vi "Get Impedance Meas Value.vi"(8 "error in (no error)":errorcluster, 11 "VISA resource name":refnum<visa-resource-name>) -> (0 "error out":errorcluster, 1 "Value Units":i32, 2 "Meas Value":dbl format="%^.3e", 3 "VISA resource name out":refnum<visa-resource-name>)   [LabVIEW 2013, in "Fluke 5XXX Series Multicalibrators.lvlib"]
doc: "This VI returns the last value of the scope impedance measurement. The unit returns indicates the status of the reading. Returns 0 and NONE when there is no recent measurement either because the Calibrator is not in a measurement mode, or because no measurement has been made yet.\n\nNote:\n\nThis VI is available only for instrument models 5500A and 5520A with oscilloscope option SC600 (SC1100)."
uses:
  Fluke 5XXX Series Multicalibrators.lvlib
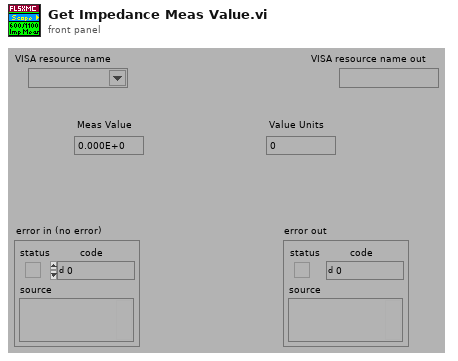
[diagram p1: front panel]
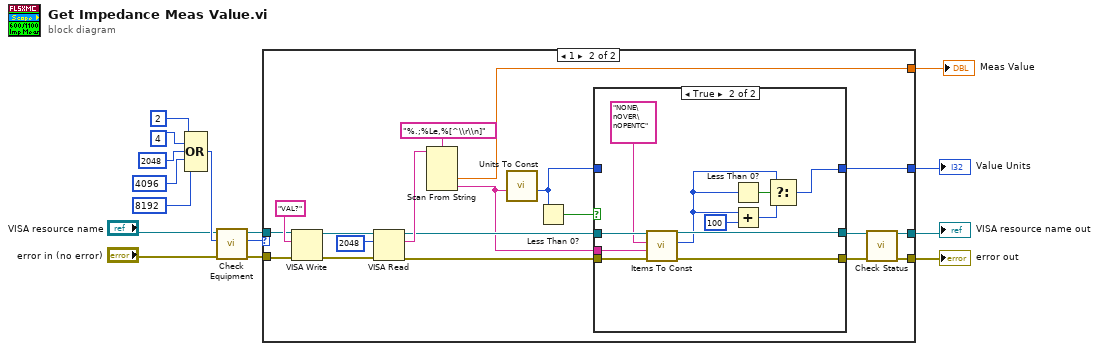
[diagram p0: block diagram]
diagram:
  n1 = Compound Arithmetic op=OR(2 ("Numeric"), 4 ("Numeric"), 2048 ("Numeric"), 4096 ("Numeric"), 8192 ("Numeric")) -> (w10:i32)
  n2 = call "Check Equipment.vi"("error in (no error)"="error in (no error)", "Bit Mask"=w10, "VISA resource name"="VISA resource name") -> ("error out"=w6:errorcluster, "Present?"=w5:u32, "VISA resource name out"=w7:refnum<visa-resource-name>)  [unwired: 6 in]
  n3 = case shown="1" w5 {
    tunnel: [w19 w33] -> w3
    tunnel: [w16 w32] -> w4
    tunnel: w6 -> [w19 w34]
    tunnel: [0.0 w29] -> w1
    tunnel: [0 w27] -> w2
    tunnel: w7 -> [w16 w21]
    frame 0, Default {
    }
    frame 1 {
      n4 = VISA Write(VISA resource name=w21, write buffer="VAL?", error in (no error)=w34) -> (VISA resource name out=w37:refnum<visa-resource-name>, error out=w36:errorcluster)  [unwired: 1 out]
      n5 = VISA Read(VISA resource name=w37, byte count=u32 2048 ("byte count (0)"), error in (no error)=w36) -> (VISA resource name out=w26:refnum<visa-resource-name>, read buffer=w30:string, error out=w23:errorcluster)  [unwired: 1 out]
      n6 = Scan From String(format string="%.;%Le,%[^\\r\\n]", input string=w30) -> (output 1=w29:dbl, output 2=w22:string)  [unwired: 4 in, 3 out]
      n7 = call "Units To Const.vi"("Units"=w22) -> ("Const"=w20:i32)  [unwired: 10 in]
      n8 = Less Than 0?(x=w20) -> (x < 0?=w28:bool)
      n9 = case shown="True" w28 {
        tunnel: w20 -> [w41 _]
        tunnel: [w41 w48] -> w27
        tunnel: w26 -> [w39 w51]
        tunnel: [w39 w52] -> w25
        tunnel: [w40 w43] -> w24
        tunnel: w23 -> [w40 w45]
        tunnel: w22 -> [_ w49]
        frame False {
        }
        frame True {
          n10 = call "Items To Const.vi"("error in (no error)"=w45, "String Item"=w49, "Multi-Line String"="NONE\nOVER\nOPENTC", "VISA resource name"=w51) -> ("error out"=w43:errorcluster, "Index"=w42:i32, "VISA resource name out"=w52:refnum<visa-resource-name>)  [unwired: 5 in]
          n11 = Less Than 0?(x=w42) -> (x < 0?=w44:bool)
          n12 = Add(x=w42, y=100) -> (x+y=w47:i32)
          n13 = Select(t=w42, s=w44, f=w47) -> (s? t:f=w48:i32)
        }
      }
      n14 = call "Check Status.vi"("VISA resource name"=w25, "error in (no error)"=w24) -> ("VISA resource name out"=w32:refnum<visa-resource-name>, "error out"=w33:errorcluster)  [unwired: 12 in]
    }
  }
  "Meas Value" <- w1
  "Value Units" <- w2
  "VISA resource name out" <- w4
  "error out" <- w3
